vi "Init Device.vi"(8 "error in (no error)":errorcluster, 11 "Virtual Camera in":refnum<class "Virtual Camera.lvclass">) -> (0 "error out":errorcluster, 3 "Virtual Camera out":refnum<class "Virtual Camera.lvclass">)   [LabVIEW 2018, in "Virtual Camera.lvlib" / "Virtual Camera.lvclass"]
uses:
  Virtual Camera.lvclass
  C:/Program Files/National Instruments/LabVIEW 2018/vi.lib/ActorFramework/Actor/Actor.lvclass
  Tiff Writer/Tiff Writer/Tiff Writer.lvclass
  Virtual Camera.lvclass/Virtual Camera.ctl
  Orca-Flash 4.0 V2/Orca-Flash 4.0 V2.lvclass
  C:/FlashGordon/Development/Hardware/Camera/Camera.lvclass
  Camera/Camera.lvclass
  <vilib>/ActorFramework/Actor/Actor.lvclass
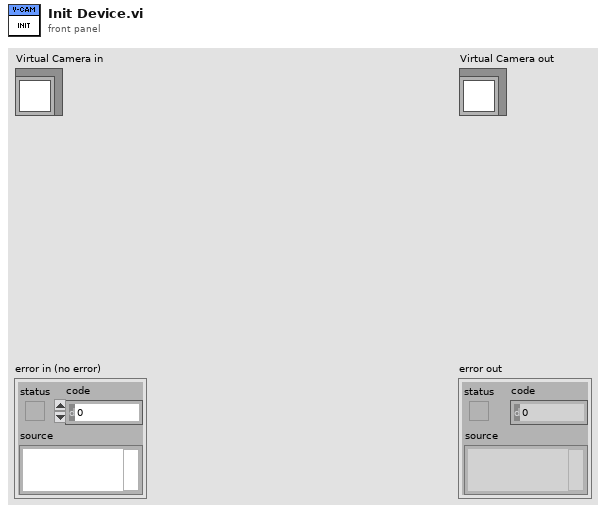
[diagram p1: front panel]
types:
  T1 = typedef "Camera Type.ctl" = enum16{"Hamamatsu"}
  T2 = typedef "Physical Camera Assignment.ctl" = cluster{"Channel Name":string, "Camera Type":T1, "Serial Number":string, "Flip Vertically":bool, "Flip Horizontally":bool, "photonsPerCount":dbl, "wavelength":i16}
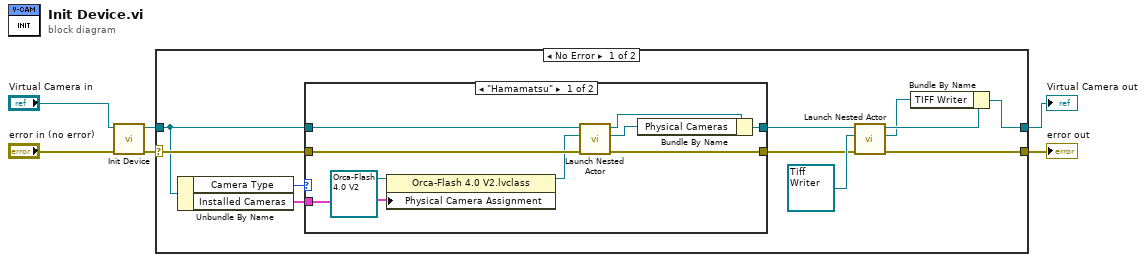
[diagram p0: block diagram]
diagram:
  n1 = call-parent "Init Device.vi"("error in (no error)"="error in (no error)", "Camera in"="Virtual Camera in") -> ("error out"=w4:errorcluster, "Camera out"=w1:refnum<class "Virtual Camera.lvclass">)  [unwired: 8 in]
  n2 = case shown="No Error" w4 {
    selector: w4 -> [w17 w30]
    tunnel: w1 -> [w16 w29]
    tunnel: [w11 w30] -> w3
    tunnel: [w8 w29] -> w2
    frame No Error {
      n3 = Unbundle By Name(w16) -> ("Camera Type"=w15:T1, "Installed Cameras"=w7:T2[])
      n4 = case shown="\"Hamamatsu\"" w15 {
        tunnel: [w25 w27] -> w12
        tunnel: [w19 w28] -> w13
        tunnel: w16 -> [w26 w28]
        tunnel: w17 -> [w24 w27]
        tunnel: w7 -> [w21 _]
        frame "Hamamatsu" {
          n5 = property class="Orca-Flash 4.0 V2.lvclass"(reference=refnum<class "Orca-Flash 4.0 V2.lvclass"> refnum ("Orca-Flash 4.0.lvlib:Orca-Flash 4.0.lvclass"), "Physical Camera Assignment"=w21) -> (reference out=w22:refnum<class "Orca-Flash 4.0 V2.lvclass">)  [unwired: 1 in, 1 out]
          n6 = call <vilib>:"Launch Nested Actor.vi"("error in (no error)"=w24, "Nested Actor"=w22, "Caller Actor in"=w26) -> ("error out"=w25:errorcluster, "Nested Actor's Enqueuer"=w18:refnum<class "Message Enqueuer.lvclass">, "Caller Actor out"=w20:refnum<class "Virtual Camera.lvclass">)  [unwired: 6 in]
          n7 = Bundle By Name(cluster=w20, "Physical Cameras"=w18) -> (w19:refnum<class "Virtual Camera.lvclass">)
        }
        frame Default {
        }
      }
      n8 = call <vilib>:"Launch Nested Actor.vi"("error in (no error)"=w12, "Nested Actor"=refnum<class "Tiff Writer.lvclass"> refnum ("Tiff Writer.lvlib:Tiff Writer.lvclass"), "Caller Actor in"=w13) -> ("error out"=w11:errorcluster, "Nested Actor's Enqueuer"=w9:refnum<class "Message Enqueuer.lvclass">, "Caller Actor out"=w10:refnum<class "Virtual Camera.lvclass">)  [unwired: 6 in]
      n9 = Bundle By Name(cluster=w10, "TIFF Writer"=w9) -> (w8:refnum<class "Virtual Camera.lvclass">)
    }
    frame Error {
    }
  }
  "error out" <- w3
  "Virtual Camera out" <- w2
